vi "Chart Send Value.vi"(8 "error in":errorcluster, 11 "Value":dbl) -> (0 "error out":errorcluster)   [LabVIEW 2014, in "Events Lib.lvlib"]
uses:
  Events Lib.lvlib
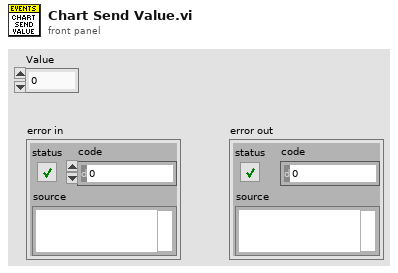
[diagram p1: front panel]
types:
  T1 = typedef "Events Lib.lvlib/Events TypeDef.ctl" = cluster{"Stop Event":refnum<user-event>, "Chart Send Value":refnum<user-event>}
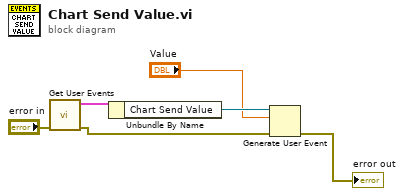
[diagram p0: block diagram]
diagram:
  n1 = call "Get User Events.vi"("error in"="error in") -> ("error out"=w1:errorcluster, "User Events Ref"=w6:T1)  [unwired: 9 in]
  n2 = Unbundle By Name(w6) -> ("Chart Send Value"=w5:refnum<user-event>)
  n3 = Generate User Event(user event=w5, event data cluster="Value", error in=w1) -> (error out=→"error out":errorcluster)  [unwired: 1 in, 1 out]
